vi "Instrument-gpib v1.0.VI"(0 "Characters to Write":string="QUERREG?2;", 1 "Write?":bool=TRUE, 2 "GPIB Address":refnum<visa-resource-name>, 3 "Timeout (msec)":i32=300 min=0 step=100, 4 "Read?":bool=TRUE) -> (5 "Error":i32 min=0 step=100, 6 "Characters Read":string="0.0;\n")   [LabVIEW 2020]
panel:
  in  "Report GPIB\nstatus/error?":bool=TRUE
  in  "Max bytes \nto read?":i32=256
  in  "Dialog box?":bool
  out "Read GPIB Error":string="No error to report"
  out "Read Status Description":string="LACS - Listener Active State\rCIC - Controller In Charge\rREM - Remote State\rCMPL - Operation Completed\rEND - EOI or EOS detected\r"
  out "Read: Byte count":i32=5
  in  "Dialog box?":bool
  out "Write GPIB Error":string="No error to report"
  out "Write Status Description":string="TACS - Talker Active State\rCIC - Controller In Charge\rREM - Remote State\rCMPL - Operation Completed\r"
  out "Write: Byte count":i32=11
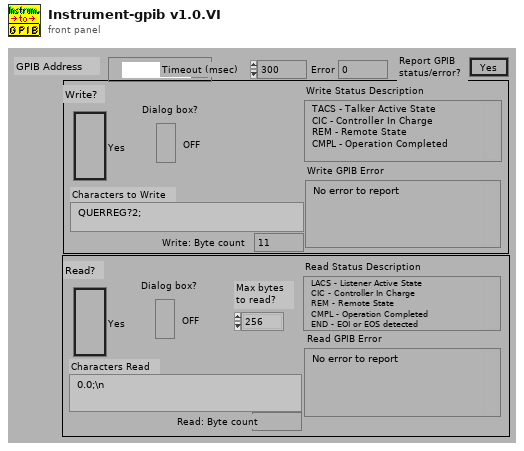
[diagram p1: front panel]
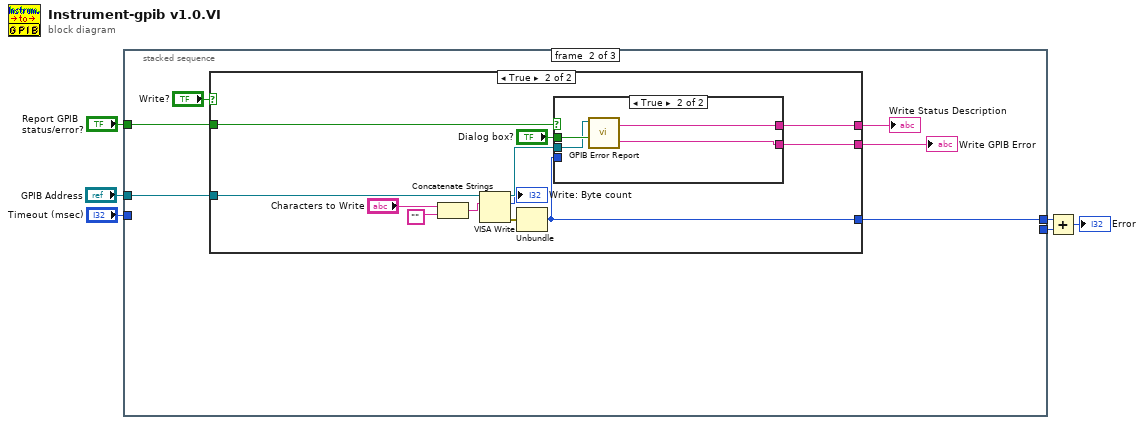
[diagram p0: block diagram]
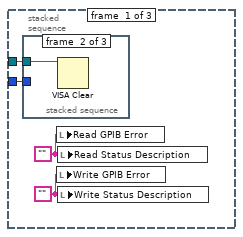
[diagram p2: hidden frame]
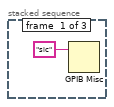
[diagram p3: hidden frame]
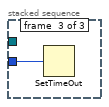
[diagram p4: hidden frame]
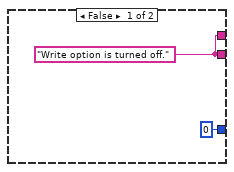
[diagram p5: hidden frame]
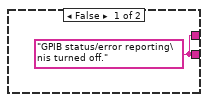
[diagram p6: hidden frame]
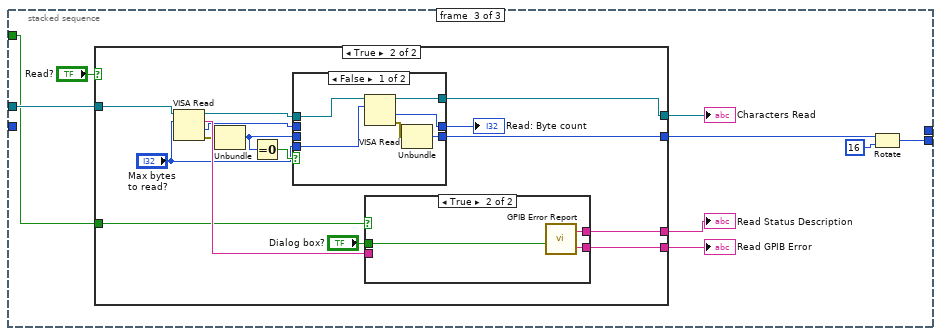
[diagram p7: hidden frame]
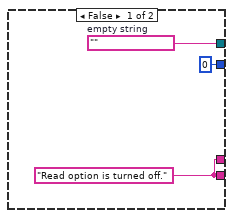
[diagram p8: hidden frame]
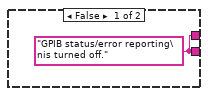
[diagram p10: hidden frame]
diagram:
  n1 = stacked-sequence {
    tunnel: "GPIB Address" -> [w7 w19 w47]
    tunnel: "Timeout (msec)" -> [w10 _ _]
    tunnel: "Report GPIB\nstatus/error?" -> [_ w18 w46]
    tunnel: [_ w14 _] -> w3
    tunnel: [_ _ w39] -> w2
    frame #0 {
      w8 = ""
      w9 = ""
      n2 = stacked-sequence {
        tunnel: w10 -> [_ _ w13]
        tunnel: w7 -> [_ w12 _]
        frame #0 {
          n3 = GPIB Misc(0:"sic") -> ()  [unwired: 1 in, 3 out]
        }
        frame #1 {
          n4 = VISA Clear(VISA resource name=w12) -> ()  [unwired: 1 in, 2 out]
        }
        frame #2 {
          n5 = SetTimeOut(1:w13) -> ()  [unwired: 1 out]
        }
      }
      n6 = local write "Read GPIB Error"(w8) -> ()
      n7 = local write "Write GPIB Error"(w9) -> ()
      n8 = local write "Read Status Description"(w8) -> ()
      n9 = local write "Write Status Description"(w9) -> ()
    }
    frame #1 {
      n10 = case shown="True" "Write?" {
        tunnel: w19 -> [_ w23]
        tunnel: [w21 w30] -> w16
        tunnel: [w21 w29] -> w15
        tunnel: w18 -> [_ w31]
        tunnel: [i16 0 w24] -> w14
        frame False {
          w21 = "Write option is turned off."
        }
        frame True {
          n11 = Concatenate Strings("Characters to Write", "") -> (w22:string)
          n12 = VISA Write(VISA resource name=w23, write buffer=w22) -> (VISA resource name out=w32:refnum<visa-resource-name>, return count=→"Write: Byte count":u32, error out=w25:errorcluster)  [unwired: 1 in]
          n13 = Unbundle(w25) -> ("code"=w24:i32)  [unwired: 2 out]
          n14 = case shown="True" w31 {
            tunnel: "Dialog box?" -> [_ w36]
            tunnel: w32 -> [_ w35]
            tunnel: w24 -> [_ _]
            tunnel: [w34 w38] -> w30
            tunnel: [w34 w37] -> w29
            frame False {
              w34 = "GPIB status/error reporting\nis turned off."
            }
            frame True {
              n15 = call "GPIB Error Report.vi"("Dialog?(F)"=w36, "Address String"=w35) -> ("Error String"=w37:string, "Status String"=w38:string)  [unwired: 2 in]
            }
          }
        }
      }
      "Write Status Description" <- w16
      "Write GPIB Error" <- w15
    }
    frame #2 {
      n16 = case shown="True" "Read?" {
        tunnel: w47 -> [_ w52]
        tunnel: [w49 w63] -> w43
        tunnel: [w49 w62] -> w42
        tunnel: [w50 w59] -> w44
        tunnel: w46 -> [_ w64]
        tunnel: [i16 0 w58] -> w41
        frame False {
          w49 = "Read option is turned off."
          w50 = ""  # empty string
        }
        frame True {
          n17 = VISA Read(VISA resource name=w52, byte count="Max bytes \nto read?") -> (VISA resource name out=w54:refnum<visa-resource-name>, read buffer=w65:string, return count=w55:u32, error out=w57:errorcluster)  [unwired: 1 in]
          n18 = Unbundle(w57) -> ("code"=w53:i32)  [unwired: 2 out]
          n19 = Equal To 0?(x=w53) -> (x = 0?=w60:bool)
          n20 = case shown="False" w60 {
            tunnel: "Max bytes \nto read?" -> [w66 _]
            tunnel: [w71 w72] -> w59
            tunnel: [w68 w74] -> w58
            tunnel: w53 -> [_ w74]
            tunnel: [w69 w73] -> w56
            tunnel: w55 -> [_ w73]
            tunnel: w54 -> [w67 w72]
            frame False {
              n21 = VISA Read(VISA resource name=w67, byte count=w66) -> (VISA resource name out=w71:refnum<visa-resource-name>, return count=w69:u32, error out=w70:errorcluster)  [unwired: 1 in, 1 out]
              n22 = Unbundle(w70) -> ("code"=w68:i32)  [unwired: 2 out]
            }
            frame True {
            }
          }
          "Read: Byte count" <- w56
          n23 = case shown="True" w64 {
            tunnel: "Dialog box?" -> [_ w76]
            tunnel: w65 -> [_ _]
            tunnel: [w75 w78] -> w63
            tunnel: [w75 w77] -> w62
            frame False {
              w75 = "GPIB status/error reporting\nis turned off."
            }
            frame True {
              n24 = call "GPIB Error Report.vi"("Dialog?(F)"=w76) -> ("Error String"=w77:string, "Status String"=w78:string)  [unwired: 3 in]
            }
          }
        }
      }
      "Characters Read" <- w44
      "Read Status Description" <- w43
      "Read GPIB Error" <- w42
      n25 = Rotate(1:16, 2:w41) -> (0:w39:i32)
    }
  }
  n26 = Add(x=w3, y=w2) -> (x+y=→"Error":i32)
